vi "error out ctl.vi"() -> (3 "error out control":string)   [LabVIEW 2013]
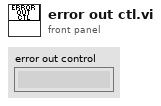
[diagram p1: front panel]
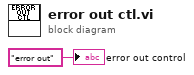
[diagram p0: block diagram]
diagram:
  "error out control" <- "error out" ("Control Name")
